vi "(SubVI) Make_card_ID.vi"() -> (0 "Card_ID":string[](array[string]))   [LabVIEW 2018]
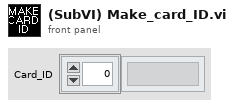
[diagram p1: front panel]
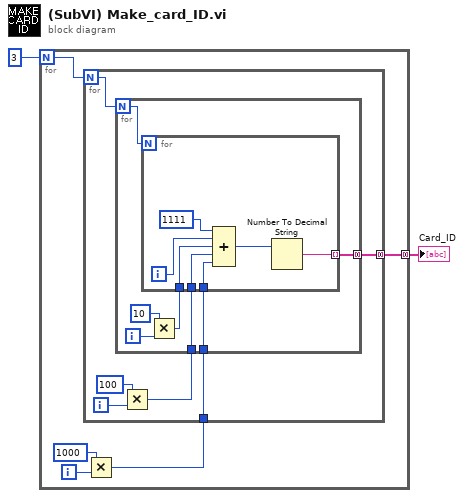
[diagram p0: block diagram]
diagram:
  n1 = for {
    N: 3 -> [w7]
    tunnel: [w3] -> w1 mode=concatenating
    i -> [w6]
    n2 = Multiply(x=1000, y=w6) -> (x*y=w4:i32)
    n3 = for {
      N: w7 -> [w13]
      tunnel: w4 -> [w9]
      tunnel: [w8] -> w3 mode=concatenating
      i -> [w11]
      n4 = Multiply(x=100, y=w11) -> (x*y=w10:i32)
      n5 = for {
        N: w13 -> [w20]
        tunnel: w10 -> [w16]
        tunnel: w9 -> [w15]
        tunnel: [w14] -> w8 mode=concatenating
        i -> [w18]
        n6 = Multiply(x=10, y=w18) -> (x*y=w17:i32)
        n7 = for {
          N: w20 -> [_]
          tunnel: w17 -> [w26]
          tunnel: w16 -> [w25]
          tunnel: w15 -> [w24]
          tunnel: [w21] -> w14 mode=indexing
          i -> [w27]
          n8 = Compound Arithmetic op=ADD(1111 ("x"), w27, w26, w25, w24) -> (w22:i32)
          n9 = Number To Decimal String(number=w22) -> (decimal integer string=w21:string)  [unwired: 1 in]
        }
      }
    }
  }
  "Card_ID" <- w1
